vi "LCR_Logfile.vi"(4 "Data Cluster":T3, 5 "Secondary Ref":refnum<vi>, 6 "Time Stamp":timestamp format="%<%x %.3X>T", 7 "Primary Ref":refnum<vi>, 8 "error in":errorcluster, 9 "Data_In":T1 {"GUI Data Cluster"."SBR" format="%08b"}, 10 "Config_In":T4={"General"={"Config.ini"=path "", "Default Logging Path"=path ""}, "Hardware"={"AHC VISA COM"="", "Measure Rate (1/s)"=0, "Global T VAR"="", "Global B VAR"="", "Average"=4, "Bias"=0, "Cable"={"Length"=0.0, "Resistance"=0.0, "Inductance"=0.0, "Capacitance"=0.0}, "Tracking"=0, "Voltage"=0.0}, "Operation"={"Operation Mode"=enum."Idle-Off", "Status"="", "NewLog?"=FALSE}}) -> (0 "error out":errorcluster, 1 "Data_Out":T1 {"GUI Data Cluster"."SBR" format="%08b"}, 2 "Config_Out":T4={"General"={"Config.ini"=path "", "Default Logging Path"=path ""}, "Hardware"={"AHC VISA COM"="", "Measure Rate (1/s)"=0, "Global T VAR"="", "Global B VAR"="", "Average"=4, "Bias"=0, "Cable"={"Length"=0.0, "Resistance"=0.0, "Inductance"=0.0, "Capacitance"=0.0}, "Tracking"=0, "Voltage"=0.0}, "Operation"={"Operation Mode"=enum."Idle-Off", "Status"="", "NewLog?"=FALSE}}, 3 "File Failure":bool)   [LabVIEW 2021]
uses:
  Config_Cluster.ctl
  Mode_Enum.ctl
  Data_Cluster.ctl
  Measurement_Cluster.ctl
panel:
  in  "Status Ref":refnum<vi>
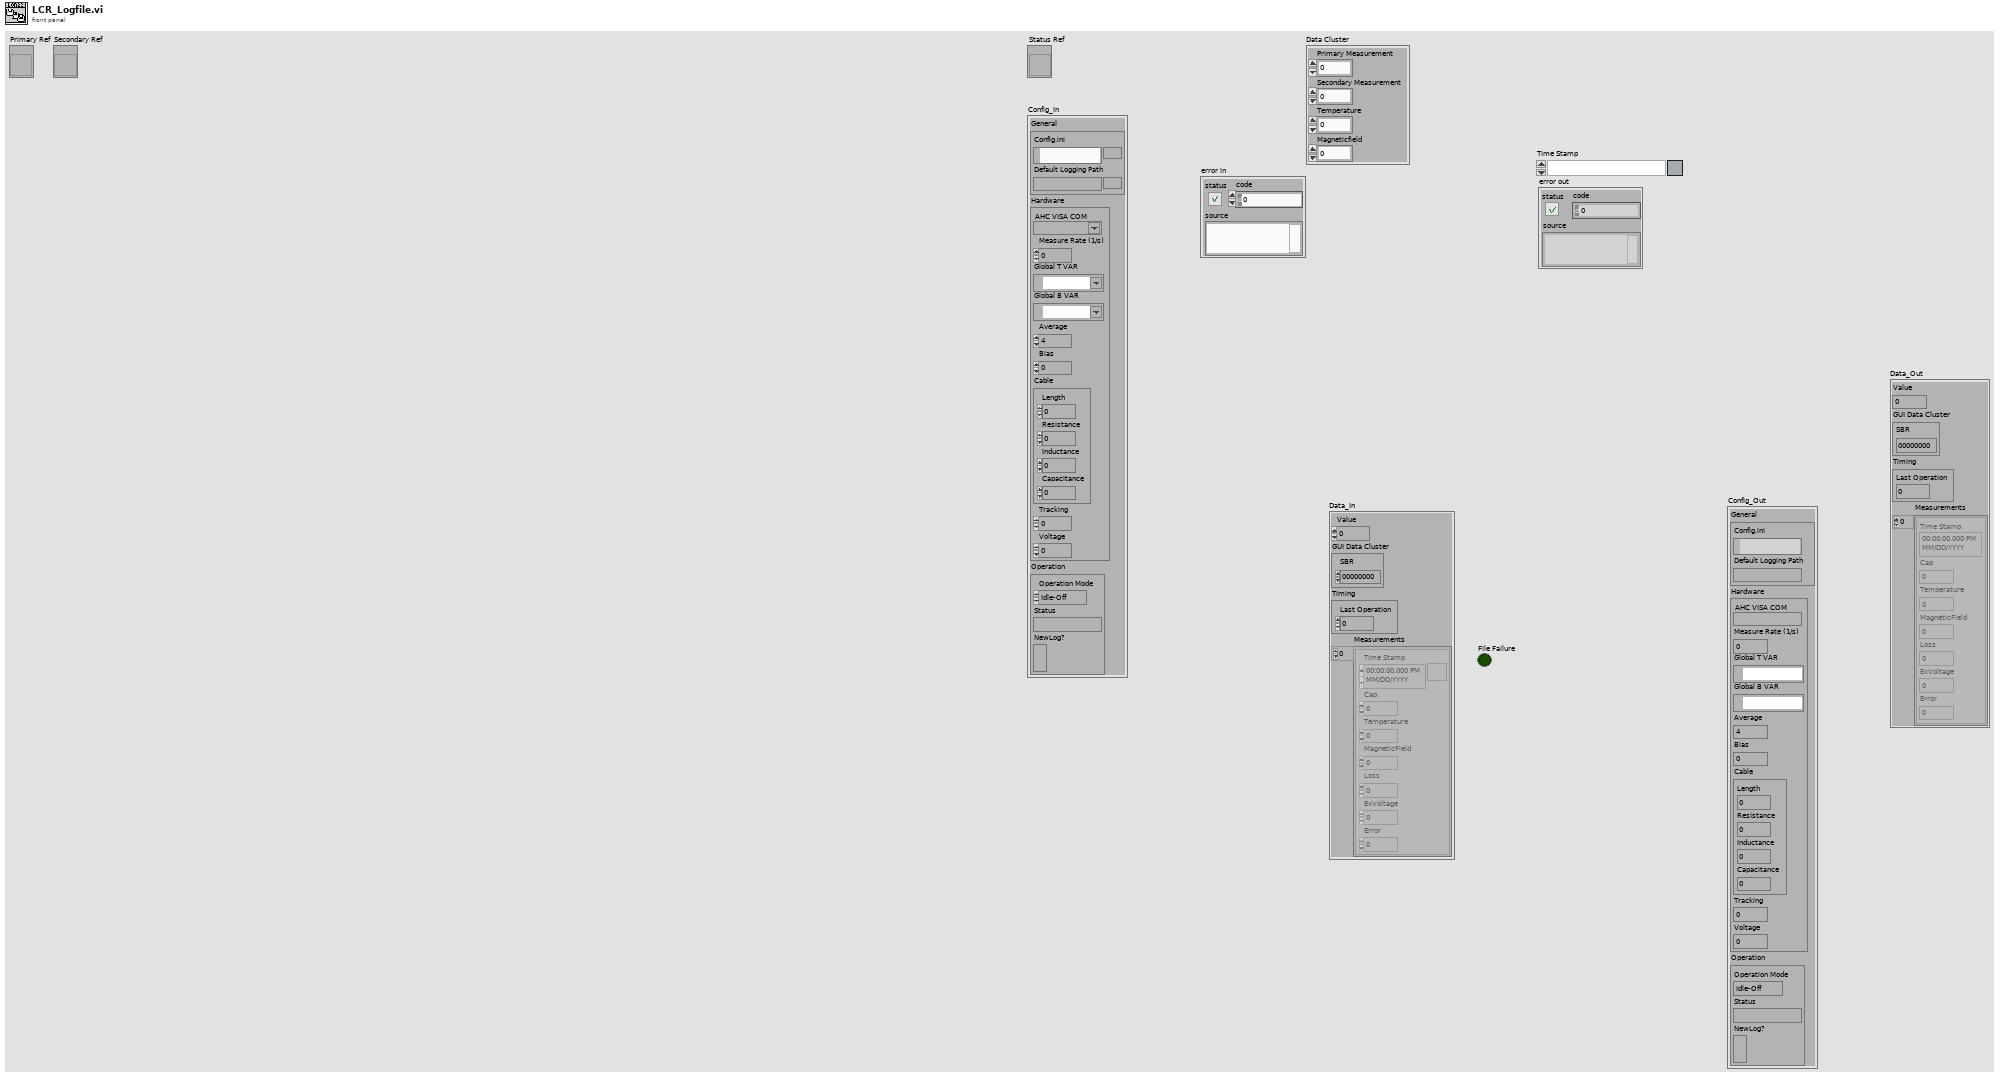
[diagram p1: front panel]
types:
  T1 = typedef "Data_Cluster.ctl" = cluster{"Value":dbl, "GUI Data Cluster":cluster{"SBR":u16}, "Timing":cluster{"Last Operation":dbl}, "Measurements":T2[]}
  T2 = typedef "Measurement_Cluster.ctl" = cluster{"Time Stamp":timestamp, "Cap":dbl, "Temperature":dbl, "MagneticField":dbl, "Loss":dbl, "ExVoltage":dbl, "Error":dbl}
  T3 = cluster{"Primary Measurement":dbl, "Secondary Measurement":dbl, "Temperature":dbl, "Magneticfield":dbl}
  T4 = typedef "Config_Cluster.ctl" = cluster{"General":cluster{"Config.ini":path, "Default Logging Path":path}, "Hardware":cluster{"AHC VISA COM":refnum<visa-resource-name>, "Measure Rate (1/s)":i32, "Global T VAR":refnum<k21>, "Global B VAR":refnum<k21>, "Average":u8, "Bias":u8, "Cable":cluster{"Length":dbl, "Resistance":dbl, "Inductance":dbl, "Capacitance":dbl}, "Tracking":u8, "Voltage":dbl}, "Operation":cluster{"Operation Mode":T5, "Status":string, "NewLog?":bool}}
  T5 = typedef "Mode_Enum.ctl" = enum16{"Logging", "Idle-Off", "Idle"}
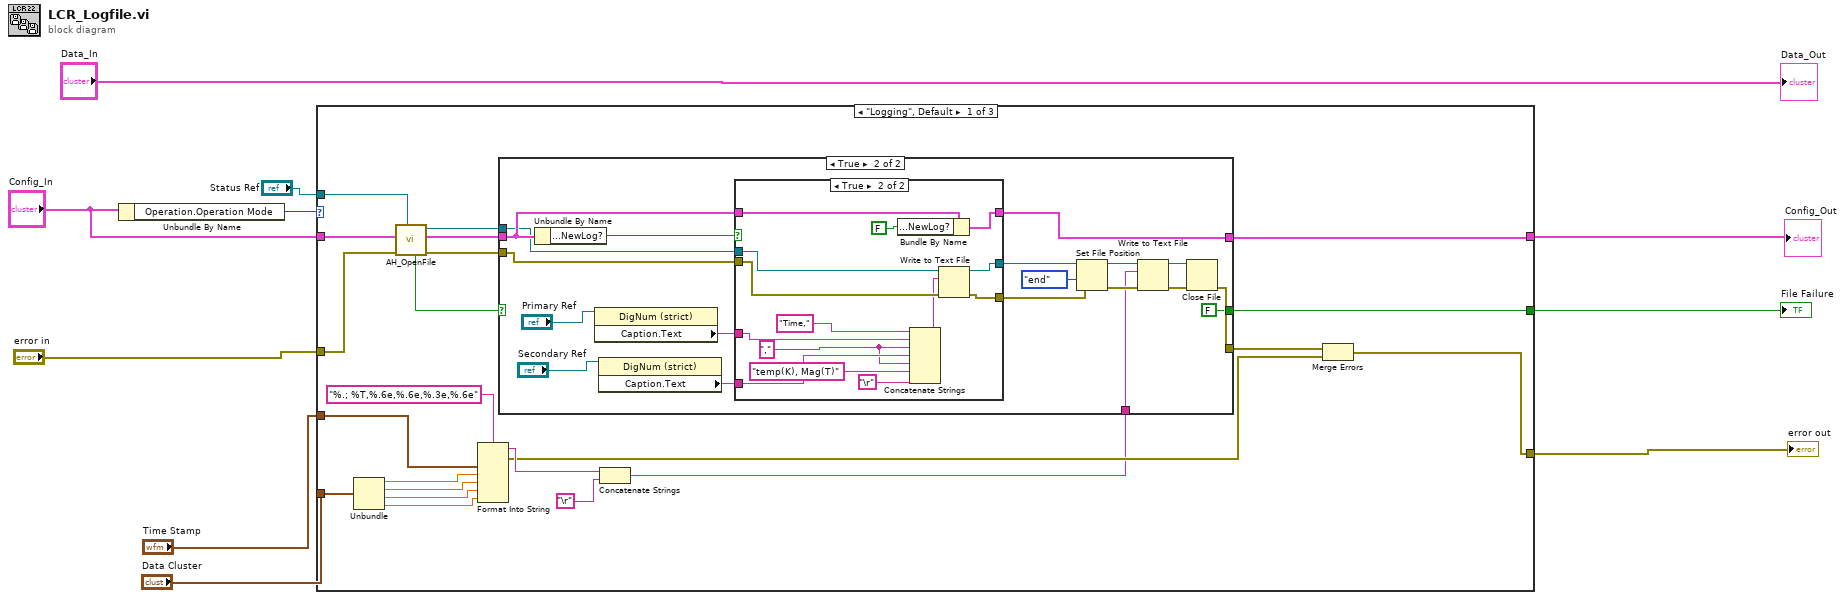
[diagram p0: block diagram]
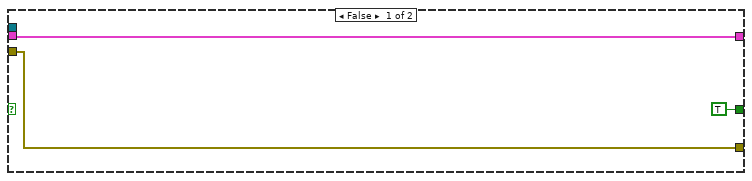
[diagram p2: hidden frame]
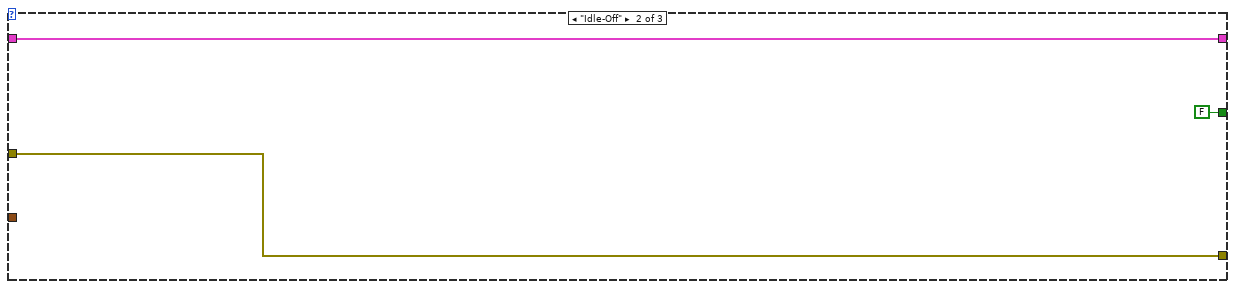
[diagram p4: hidden frame]
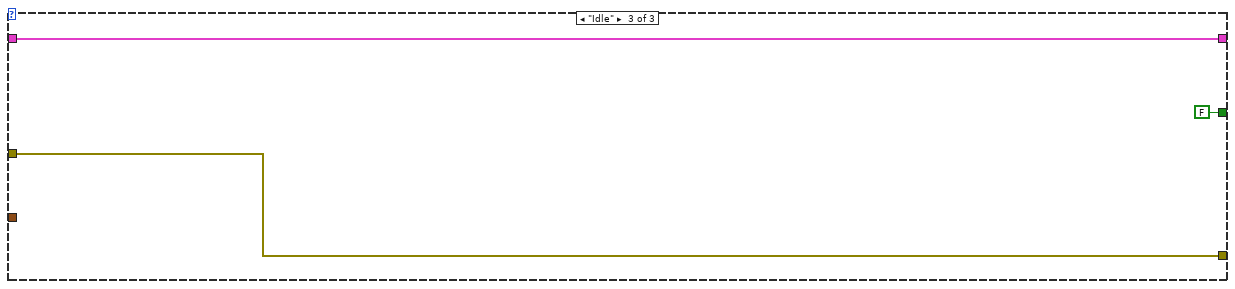
[diagram p5: hidden frame]
diagram:
  n1 = Unbundle By Name("Config_In") -> ("Operation.Operation Mode"=w6:T5)
  n2 = case shown="\"Logging\", Default" w6 {
    tunnel: "error in" -> [w21 w74 w77]
    tunnel: "Time Stamp" -> [w31 _ _]
    tunnel: [w13 w74 w77] -> w9
    tunnel: "Data Cluster" -> [w26 _ _]
    tunnel: "Config_In" -> [w23 w73 w76]
    tunnel: "Status Ref" -> [w22 _ _]
    tunnel: [w12 w73 w76] -> w2
    tunnel: [w11 FALSE FALSE] -> w1
    frame "Logging", Default {
      n3 = Unbundle(w26) -> ("Primary Measurement"=w30:dbl, "Secondary Measurement"=w29:dbl, "Temperature"=w28:dbl, "Magneticfield"=w27:dbl)
      n4 = call "AH_OpenFile.vi"("Status Ref"=w22, "error in"=w21, "Config_Cluster"=w23) -> ("error out"=w17:errorcluster, "Config_Cluster Out"=w18:T4, "refnum out"=w19:refnum<file>, "FileOpen?"=w20:bool)  [unwired: 5 in]
      n5 = Format Into String(format string="%.; %T,%.6e,%.6e,%.3e,%.6e", w31, w30, w29, w28, w27) -> (resulting string=w25:string, error out=w16:errorcluster)  [unwired: 2 in]
      n6 = Concatenate Strings(w25, "\r") -> (w15:string)
      n7 = case shown="True" w20 {
        tunnel: w19 -> [_ w44]
        tunnel: w18 -> [w34 w46]
        tunnel: w17 -> [w35 w43]
        tunnel: w15 -> [_ w48]
        tunnel: [w35 w47] -> w14
        tunnel: [w34 w45] -> w12
        tunnel: [TRUE FALSE] -> w11
        frame False {
        }
        frame True {
          n8 = Unbundle By Name(w46) -> ("Operation.NewLog?"=w54:bool)
          n9 = property class="DigNum (strict)"(reference="Primary Ref") -> ("Caption.Text"=w38:string)  [unwired: 1 in, 2 out]
          n10 = property class="DigNum (strict)"(reference="Secondary Ref") -> ("Caption.Text"=w37:string)  [unwired: 1 in, 2 out]
          n11 = case shown="True" w54 {
            tunnel: w46 -> [w57 w71]
            tunnel: [w57 w70] -> w45
            tunnel: w44 -> [w56 w66]
            tunnel: w43 -> [w55 w65]
            tunnel: [w56 w68] -> w42
            tunnel: [w55 w67] -> w41
            tunnel: w38 -> [_ w63]
            tunnel: w37 -> [_ w62]
            frame False {
            }
            frame True {
              w61 = "," ("string")
              n12 = Bundle By Name(cluster=w71, "Operation.NewLog?"=FALSE) -> (w70:T4)
              n13 = Concatenate Strings("Time,", w63, w61, w62, w61, "temp(K), Mag(T)" ("string"), "\r") -> (w58:string)
              n14 = Write to Text File(file (use dialog)=w66, text=w58, error in=w65) -> (refnum out=w68:refnum<file>, error out=w67:errorcluster)  [unwired: 1 in, 1 out]
            }
          }
          n15 = Set File Position(refnum=w42, from (0:start)=enum16{"start", "end", "current"}."end", error in=w41) -> (refnum out=w52:refnum<file>, error out=w53:errorcluster)  [unwired: 1 in]
          n16 = Write to Text File(file (use dialog)=w52, text=w48, error in=w53) -> (refnum out=w51:refnum<file>, error out=w50:errorcluster)  [unwired: 1 in, 1 out]
          n17 = Close File(refnum=w51, error in=w50) -> (error out=w47:errorcluster)  [unwired: 1 out]
        }
      }
      n18 = Merge Errors(w14, w16) -> (w13:errorcluster)
    }
    frame "Idle-Off" {
    }
    frame "Idle" {
    }
  }
  "error out" <- w9
  "Config_Out" <- w2
  "File Failure" <- w1
  "Data_Out" <- "Data_In"
